vi "ER2007 Are You Sure Popup Panel.vi"() -> ()   [LabVIEW 2013]
uses:
  Controls/Global ER2007.vi
panel:
  in  "Cancel":bool
  in  "OK":bool
  # "Are you sure you want to Stop ?"
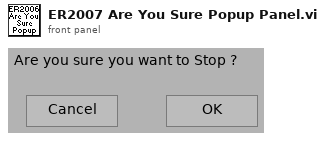
[diagram p1: front panel]
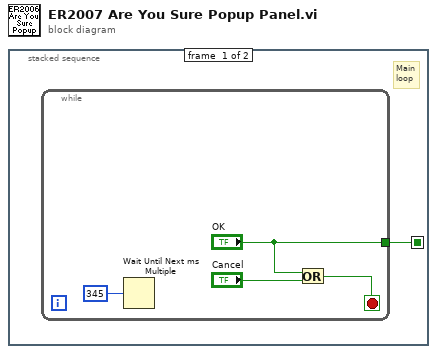
[diagram p0: block diagram]
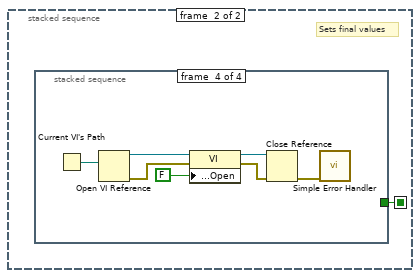
[diagram p2: hidden frame]
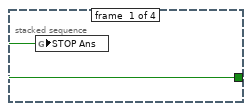
[diagram p3: hidden frame]
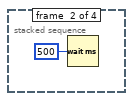
[diagram p4: hidden frame]
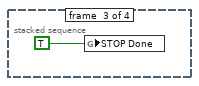
[diagram p5: hidden frame]
diagram:
  n1 = stacked-sequence {
    seq-local: [w1 _] -> [_ w6]
    frame #0 {
      # "Main\nloop"
      n2 = while {
        tunnel: ["OK"] -> w1
        stop <- w3 stop-if-true
        n3 = Wait Until Next ms Multiple(millisecond multiple=u32 345) -> ()  [unwired: 1 out]
        n4 = Or(x="OK", y="Cancel") -> (x .or. y?=w3:bool)
      }
    }
    frame #1 {
      # "Sets final values"
      n5 = stacked-sequence {
        tunnel: w6 -> [w7 _ _ _]
        frame #0 {
          n6 = global write "Global ER2007.vi" "STOP Ans"(w7) -> ()
        }
        frame #1 {
          n7 = Wait (ms)(milliseconds to wait=u32 500) -> ()  [unwired: 1 out]
        }
        frame #2 {
          n8 = global write "Global ER2007.vi" "STOP Done"(TRUE ("STOP Done")) -> ()
        }
        frame #3 {
          n9 = Current VI's Path() -> (path=w16:path)
          n10 = Open VI Reference(vi path=w16) -> (vi reference=w15:refnum<vi>, error out=w14:errorcluster)  [unwired: 5 in]
          n11 = property class="VI"(reference=w15, error in=w14, "Front Panel Window:Open"=FALSE) -> (reference out=w12:refnum<vi>, error out=w11:errorcluster)
          n12 = Close Reference(reference=w12, error in (no error)=w11) -> (error out=w10:errorcluster)
          n13 = call <vilib>:"Simple Error Handler.vi"("error in (no error)"=w10) -> ()  [unwired: 4 in, 5 out]
        }
      }
    }
  }
